vi "101-3102-report1p1-gaydos.vi"() -> ()   [LabVIEW 2012]
panel:
  out "Variance":dbl
  out "Mean":dbl
  out "Waveform Graph":dbl[](graph)
  in  "Amount of Elements":dbl
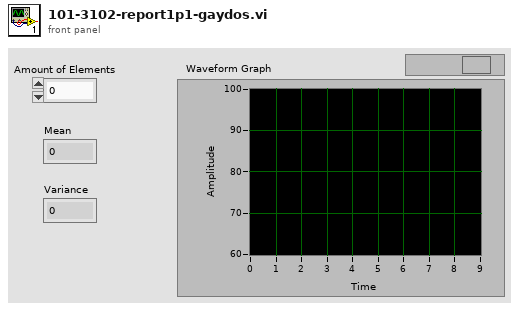
[diagram p1: front panel]
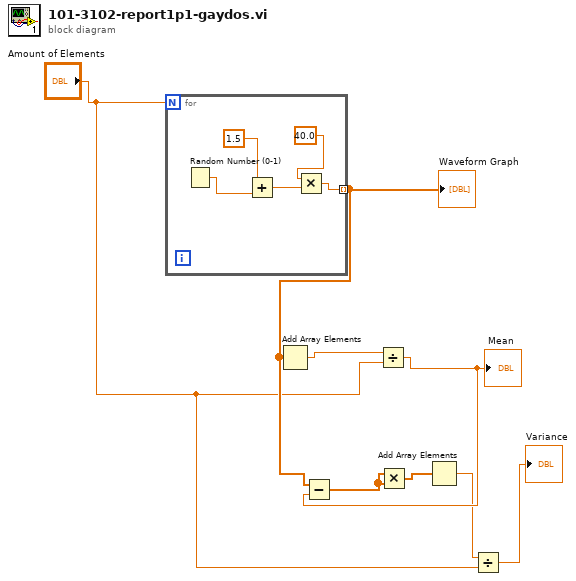
[diagram p0: block diagram]
diagram:
  n1 = for {
    N: "Amount of Elements" -> [_]
    tunnel: [w9] -> w7 mode=indexing
    n2 = Random Number (0-1)() -> (number: 0 to 1=w12:dbl)
    n3 = Add(x=1.5, y=w12) -> (x+y=w11:dbl)
    n4 = Multiply(x=40.0, y=w11) -> (x*y=w9:dbl)
  }
  "Waveform Graph" <- w7
  n5 = Add Array Elements(numeric array=w7) -> (sum=w8:dbl)
  n6 = Divide(x=w8, y="Amount of Elements") -> (x/y=w6:dbl)
  "Mean" <- w6
  n7 = Subtract(x=w7, y=w6) -> (x-y=w5:dbl[])
  n8 = Multiply(x=w5, y=w5) -> (x*y=w4:dbl[])
  n9 = Add Array Elements(numeric array=w4) -> (sum=w3:dbl)
  n10 = Divide(x=w3, y="Amount of Elements") -> (x/y=→"Variance":dbl)
